vi "로컬변수 실습.vi"() -> ()   [LabVIEW 2020]
panel:
  in  "정지":bool
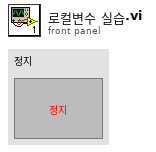
[diagram p1: front panel]
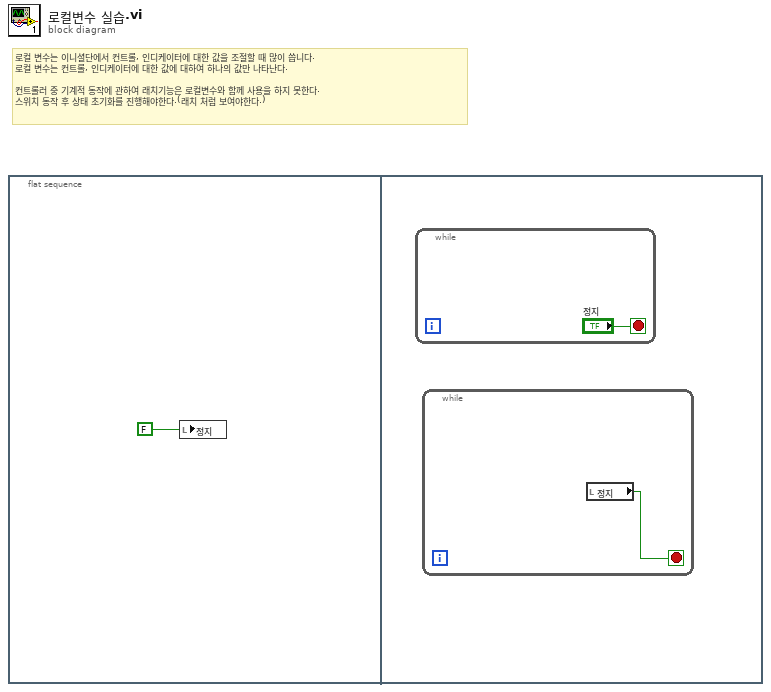
[diagram p0: block diagram]
diagram:
  # "로컬 변수는 이니셜단에서 컨트롤, 인디케이터에 대한 값을 조절할 때 많이 씁니다.\n로컬 변수는 컨트롤, 인디케이터에 대한 값에 대하여 하나의 값만 나타난다.\n\n컨트롤러 중 기계적 동작에 관하여 래치기능은 로컬변수와 함께 사용을 하지 못한다.\n스위치 동작 후 상태 초기화를 진행해야한다.(래치 처럼 보여야한다.)"
  n1 = flat-sequence {
    frame #0 {
      n2 = local write "정지"(FALSE) -> ()
    }
    frame #1 {
      n3 = while {
        stop <- "정지" stop-if-true
      }
      n4 = while {
        stop <- w2 stop-if-true
        n5 = local read "정지"() -> (w2:bool)
      }
    }
  }
